vi "Register gRPC Methods.vi"(8 "error in (no error)":errorcluster, 11 "Template Server in":refnum<class "Streamer_server.lvclass">) -> (0 "error out":errorcluster, 3 "Template Server out":refnum<class "Streamer_server.lvclass">)   [LabVIEW 2019, in "Streamer_server.lvlib" / "Streamer_server.lvclass"]
uses:
  Streamer_server.lvclass
  typeDefs/Server Internal UEs.ctl
  typeDefs/Server Internal Message.ctl
  typeDefs/Server gRPC UEs.ctl
  <vilib>/gRPC/LabVIEW gRPC Library/Server API/typeDefs/gRPCId Cluster.ctl
  <vilib>/gRPC/LabVIEW gRPC Library/Server API/typeDefs/grpcId.ctl
  Streamer_server.lvclass/Streamer_server.ctl
  <vilib>/gRPC/LabVIEW gRPC Library/gprc-lvsupport-release.lvlib
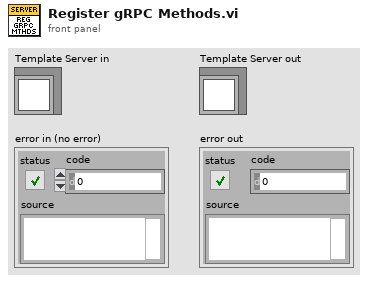
[diagram p1: front panel]
types:
  T1 = typedef "Streamer_server.lvlib/Streamer_server.lvclass/Server gRPC UEs.ctl" = cluster{"SignalStreamer_GetDataStream gRPC UE":refnum<user-event>}
  T2 = typedef "Streamer_server.lvlib/Streamer_server.lvclass/Server Internal UEs.ctl" = cluster{"SignalStreamer_GetDataStream Internal UE":refnum<user-event>}
  T3 = typedef "gprc-lvsupport-release.lvlib/grpcId.ctl" = u64
  T4 = typedef "Streamer_server.lvlib/Streamer_server.lvclass/Server Internal Message UE.ctl" = refnum<user-event>
  T5 = typedef "gprc-lvsupport-release.lvlib/gRPCId Cluster UE.ctl" = refnum<user-event>
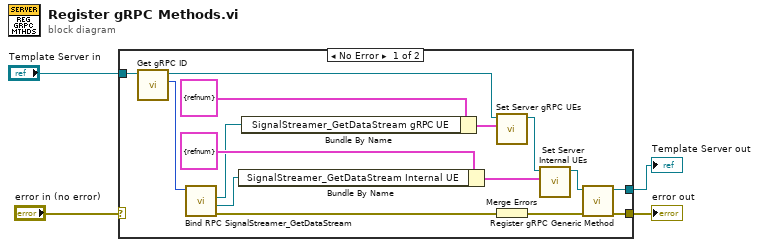
[diagram p0: block diagram]
diagram:
  n1 = case shown="No Error" "error in (no error)" {
    selector: "error in (no error)" -> [_ w20]
    tunnel: "Template Server in" -> [w18 w21]
    tunnel: [w11 w20] -> w3
    tunnel: [w9 w21] -> w2
    frame No Error {
      n2 = call "Get gRPC ID.vi"("OOP Server in"=w18) -> ("gRPC ID"=w8:T3, "OOP Server out"=w19:refnum<class "Streamer_server.lvclass">)  [unwired: 9 in]
      n3 = call "Bind RPC SignalStreamer_GetDataStream.vi"("gRPCid server in"=w8) -> ("error out"=w7:errorcluster, "SignalStreamer_GetDataStream Internal UE"=w5:T4, "SignalStreamer_GetDataStream gRPC UE"=w6:T5)  [unwired: 7 in, 1 out]
      n4 = Bundle By Name ("Bundle Internal UEs")(cluster=T2 {"SignalStreamer_GetDataStream Internal UE"=refnum} ("Server Internal UEs"), "SignalStreamer_GetDataStream Internal UE"=w5) -> (w17:T2)
      n5 = Bundle By Name ("Bundle gRPC UEs")(cluster=T1 {"SignalStreamer_GetDataStream gRPC UE"=refnum} ("gRPC Server Method Events"), "SignalStreamer_GetDataStream gRPC UE"=w6) -> (w14:T1)
      n6 = call "Set Server gRPC UEs.vi"("Server RPC Methods"=w14, "OOP Server in"=w19) -> ("OOP Server out"=w15:refnum<class "Streamer_server.lvclass">)  [unwired: 9 in]
      n7 = Merge Errors(w7) -> (w12:errorcluster)
      n8 = call "Set Server Internal UEs.vi"("Server Internal UEs"=w17, "OOP Server in"=w15) -> ("OOP Server out"=w10:refnum<class "Streamer_server.lvclass">)  [unwired: 9 in]
      n9 = call "Register gRPC Generic Method.vi"("error in (no error)"=w12, "Template Server in"=w10) -> ("error out"=w11:errorcluster, "Template Server out"=w9:refnum<class "Streamer_server.lvclass">)  [unwired: 8 in]
    }
    frame Error {
    }
  }
  "error out" <- w3
  "Template Server out" <- w2
